vi "MPUSBGetDLLVersion.vi"(8 "error in (no error)":errorcluster) -> (0 "error out":errorcluster, 2 "DLLver":string, 3 "return type":u32 format="%08x")   [LabVIEW 2019]
doc: "// MPUSBGetDLLVersion : get mpusbapi.dll revision level\n//\n// Input:\n// None\n// Output:\n// 32-bit revision level MMmmddii\n// MM - Major release\n// mm - Minor release\n// dd - dot release or minor fix\n// ii - test release revisions\n\nWritten by: Complete Automated Solutions\nwww.CompleteAutomatedSolutions.com"
uses:
  mpusbapi.dll
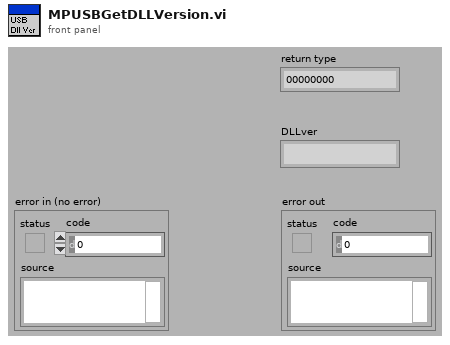
[diagram p1: front panel]
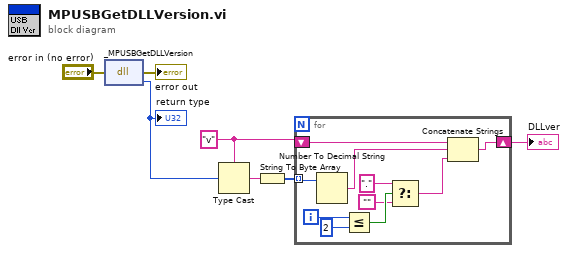
[diagram p0: block diagram]
diagram:
  w3 = "v"
  n1 = dll-call lib="C:/Users/z003r4zd/Desktop/Point Contact Mods 2019/Automation/Actuonix/LAC+Labview+Example/Actuonix_LAC_LabVIEW_Example/USB_VIs/mpusbapi.dll" fn="_MPUSBGetDLLVersion"(error in="error in (no error)") -> (error out=→"error out":errorcluster, "return type"=w4:u32)  [unwired: 2 in, 1 out]
  "return type" <- w4
  n2 = Type Cast(type=w3, x=w4) -> (*(type *) &x=w2:string)
  n3 = String To Byte Array(string=w2) -> (unsigned byte array=w1:u8[])
  n4 = for {
    shift-right: [w16] -> w5
    shift-left: w3 -> [w17]
    tunnel: w1 -> [w15] mode=indexing
    i -> [w13]
    n5 = Number To Decimal String(number=w15) -> (decimal integer string=w14:string)  [unwired: 1 out]
    n6 = Less Or Equal?(x=w13, y=2) -> (x <= y?=w10:bool)
    n7 = Select(t="." ("string"), s=w10, f="") -> (s? t:f=w8:string)
    n8 = Concatenate Strings(w17, w14, w8) -> (w16:string)
  }
  "DLLver" <- w5
